vi "读取.vi"(6 "测试人员":string, 8 "error in (no error)":errorcluster, 11 "db file":path=path "D:/Data/样品标记.sqlite3") -> (0 "error out":errorcluster, 4 "样品标记":string[](array[string]))   [LabVIEW 2020]
uses:
  <vilib>/drjdpowell/SQLite Library/SQL Connection/Open (path).vi
  <vilib>/drjdpowell/SQLite Library/SQL Connection/Open (string).vi
  <vilib>/AdvancedString/Path To Command Line String.vi
  <vilib>/drjdpowell/SQLite Library/SQL Connection/Execute SQL (1D String).vi
  <vilib>/drjdpowell/SQLite Library/SQL Connection/Connection.lvclass
  <vilib>/drjdpowell/SQLite Library/SQLite.lvlib
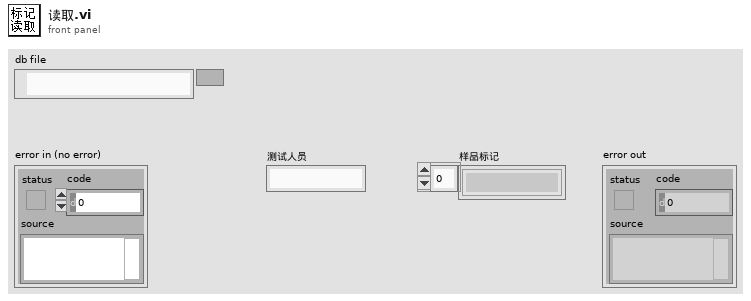
[diagram p1: front panel]
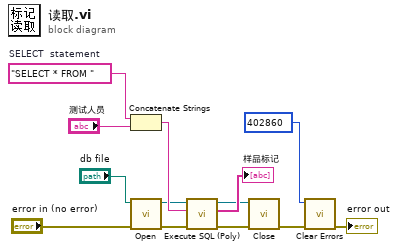
[diagram p0: block diagram]
diagram:
  w12 = "SELECT * FROM "  # SELECT  statement
  n1 = Concatenate Strings(w12, "测试人员") -> (w8:string)
  n2 = call-poly <vilib>:"Open.vi"("error in (no error)"="error in (no error)", "db file"="db file") -> ("error out"=w5:errorcluster, "SQLite Connection"=w6:refnum<class "Connection.lvclass">)  [unwired: 8 in]
  n3 = call-poly <vilib>:"Execute SQL (Poly).vi"("error in (no error)"=w5, "SQL"=w8, "SQLite Connection in"=w6) -> ("error out"=w4:errorcluster, "Result Set"=→"样品标记":string[], "SQLite Connection"=w3:refnum<class "Connection.lvclass">)  [unwired: 5 in, 1 out]
  n4 = call-dynamic "Close.vi"("error in (no error)"=w4, "SQLite Connection in"=w3) -> ("error out"=w9:errorcluster)  [unwired: 9 in]
  n5 = call <vilib>:"Clear Errors.vi"("error in (no error)"=w9, "specific error code to clear (0: all)"=402860) -> ("error out"=→"error out":errorcluster)  [unwired: 4 in, 1 out]
